vi "S8300E_SATA_HDD_Model_WIH.vi"() -> ()   [LabVIEW 2011]
panel:
  out "PRELOG2":string
  out "PRELOG1":string
  out "SATA_HDD_NUM":string
  out "CMDList":cluster{string, string, string}[](array[cluster])
  out "log msg":string
  out "VISA resource name out":refnum<visa-resource-name>
  out "BEGIN TIME":u32
  out "進行狀況":string
  # "2015-6-1"
  # "S8300E SATA  HDD Model Test(接UART COM9)"
  # "Error Code:SATA-HDD"
  # "Please insert the correct HDD Drive for Shipment\n請插入正確的出貨硬碟 (Model numer 需正確輸入於特定文檔)"
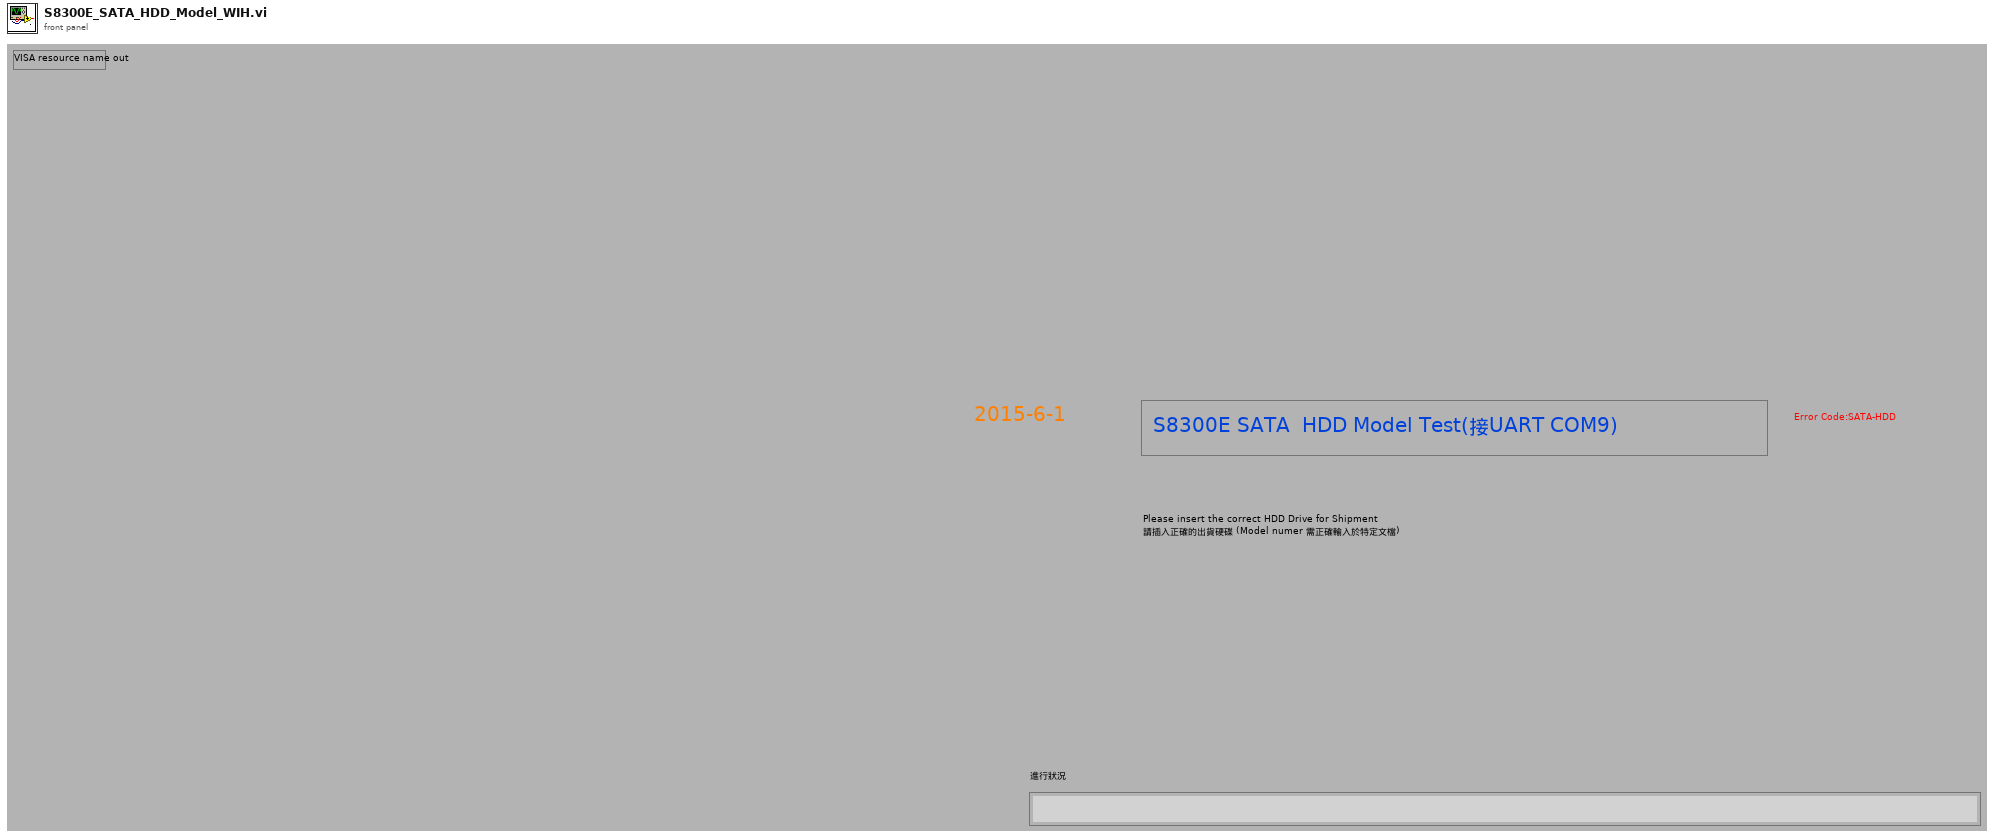
[diagram p1: front panel]
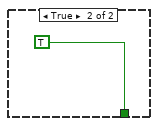
[diagram p7: hidden frame]
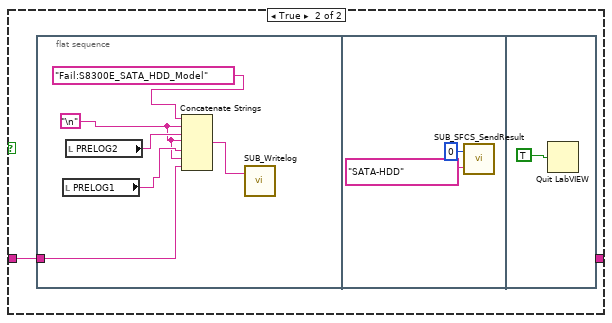
[diagram p8: hidden frame]
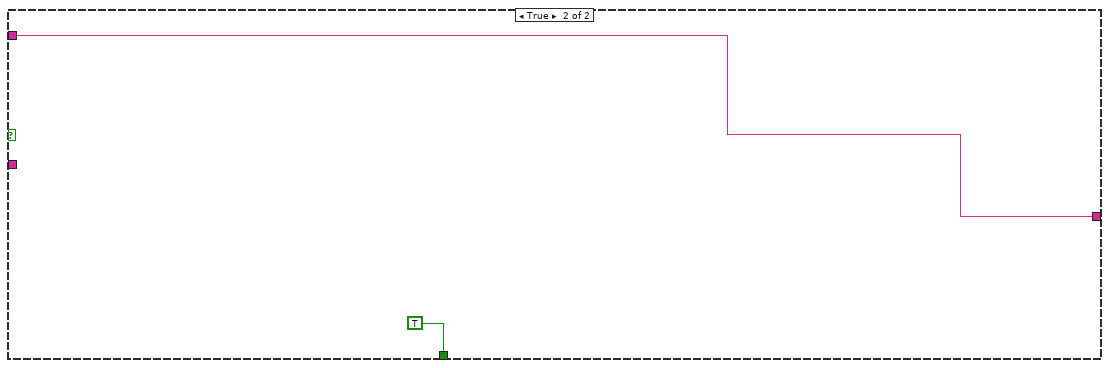
[diagram p9: hidden frame]
diagram:
  n1 = flat-sequence {
    frame #0 {
      n2 = Tick Count (ms)() -> (millisecond timer value=→"BEGIN TIME":u32)
    }
    frame #1 {
      n3 = property on="進行狀況" class="Str"("Blinking"=TRUE) -> ()  [unwired: 2 in, 2 out]
      "進行狀況" <- "進入測試準備中...." ("進行狀況")
    }
    frame #2 {
      n4 = call "SUB_SearchFile_inFolder.vi"("Search Filename in Folder"="S8300E_sfcs_misc.txt") -> ("File Existing True/Flase"=w4:bool)  [unwired: 1 in]
      n5 = case shown="False" w4 {
        frame False {
          n6 = flat-sequence {
            frame #0 {
              n7 = call "Display Message to User"() -> ()  [unwired: 10 in, 2 out]
            }
            frame #1 {
              n8 = call "SUB_Writelog.vi"("Pass/Fail"="Fail:S8300E_SATA_HDD_Model") -> ()  [unwired: 2 in]
            }
            frame #2 {
              n9 = Quit LabVIEW(quit? (T)=TRUE) -> ()
            }
          }
        }
        frame True {
        }
      }
    }
    frame #3 {
      n10 = call "SUB_Read_specifFile.vi"("name or relative path"="S8300E_sfcs_misc.txt" ("Search Filename in Folder")) -> ("text"=w11:string)  [unwired: 1 in, 1 out]
      n11 = call "SUB_FindSpecificString.vi"("Find this String"="UUT_SATA_HDD_MODEL=", "String data"=w11) -> ("before \"; \" string"=→"SATA_HDD_NUM":string, "Found"=w9:bool)  [unwired: 2 in]
      n12 = case shown="False" w9 {
        frame False {
          n13 = flat-sequence {
            frame #0 {
              n14 = call "Display Message to User2"() -> ()  [unwired: 10 in, 2 out]
            }
            frame #1 {
              n15 = call "SUB_Writelog.vi"("Pass/Fail"="Fail:S8300E_SATA_HDD_Model") -> ()  [unwired: 2 in]
            }
            frame #2 {
              n16 = Quit LabVIEW(quit? (T)=TRUE) -> ()
            }
          }
        }
        frame True {
        }
      }
    }
    frame #4 {
      n17 = local read "SATA_HDD_NUM"() -> (w16:string)
      n18 = Concatenate Strings("PASSED=", w16) -> (w15:string)
      n19 = Concatenate Strings("./sata.sh -m 1", "\r") -> (w21:string)
      n20 = Bundle(w21, w15, "Checking SATA  HDD Mdel Number") -> (w19:cluster{string, string, string})  [unwired: 1 in]
      n21 = Build Array(w19) -> (→"CMDList":cluster{string, string, string}[])
    }
    frame #5 {
      n22 = call "SUB_COM1_CLOSE.vi"("VISA resource name"=refnum<visa-resource-name> "COM9") -> ()  [unwired: 3 in]
    }
    frame #6 {
      n23 = case shown="True" TRUE {
        frame False {
        }
        frame True {
          n24 = call "SUB_COM9_INIT.vi"("baud rate"=u32 115200) -> ("VISA resource name out"=w29:refnum<visa-resource-name>)  [unwired: 1 in, 1 out]
          "VISA resource name out" <- w29
          n25 = call "SUB_COM1Wrt.vi"("VISA resource name"=w29, "write buffer"="\r") -> ("duplicate VISA resource name"=w26:refnum<visa-resource-name>)  [unwired: 1 in, 1 out]
          n26 = call "SUB_ContinueCom1Read.vi"("Numeric"=1200, "duplicate VISA resource name 2"=w26) -> ()  [unwired: 1 in, 3 out]
        }
      }
    }
    frame #7 {
      n27 = case shown="True" TRUE {
        frame False {
        }
        frame True {
          n28 = while {
            stop <- w41 stop-if-true
            n29 = local read "VISA resource name out"() -> (w32:refnum<visa-resource-name>)
            n30 = call "SUB_ContinueCom1Read.vi"("Numeric"=1200, "duplicate VISA resource name 2"=w32) -> ("duplicate VISA resource name"=w33:refnum<visa-resource-name>)  [unwired: 1 in, 2 out]
            n31 = call "SUB_COM1Wrt.vi"("VISA resource name"=w33, "write buffer"="\r") -> ("duplicate VISA resource name"=w40:refnum<visa-resource-name>)  [unwired: 1 in, 1 out]
            n32 = Tick Count (ms)() -> (millisecond timer value=w39:u32)
            n33 = call "SUB_READ_COM1_FindString_timeout.vi"("Find this String"="s8300e_func_test#", "Timeout Seccond"=3.0, "Begin time"=w39, "duplicate VISA resource name 2"=w40) -> ("Output String"=w35:string, "Found String"=w36:bool)  [unwired: 1 in, 1 out]
            n34 = case shown="False" w36 {
              tunnel: [w47 TRUE] -> w41
              tunnel: w35 -> [w44 _]
              frame False {
                w46 = "UART無正確反應!需有S8300E字串" ("Status")
                n35 = call "SUB_YESNO.vi"("Debug View"=w44, "Status"=w46) -> ("yes/no"=w50:enum32{"No Selection", "Yes", "No", "None"})  [unwired: 1 in]
                n36 = Concatenate Strings(w46, "\n", w44) -> (w43:string)
                n37 = Equal?(x=w50, y=enum32{"No Selection", "Yes", "No", "None"}."No") -> (x = y?=w48:bool)
                n38 = case shown="True" w48 {
                  tunnel: [_ w52] -> w47
                  tunnel: w43 -> [_ w51]
                  frame False {
                  }
                  frame True {
                    n39 = flat-sequence {
                      tunnel: w51 -> [w54]
                      tunnel: [w59] -> w52
                      frame #0 {
                        n40 = Concatenate Strings("Fail:S8300E_SATA_HDD_Model" ("Pass/Fail"), "\n", w54) -> (w53:string)
                        n41 = call "SUB_Writelog.vi"("Pass/Fail"=w53) -> ()  [unwired: 2 in]
                      }
                      frame #1 {
                        n42 = call "SUB_SFCS_SendResult.vi"("ErrorCode"="UART", "PASS_Fail (1/0)"=i8 0) -> ()  [unwired: 1 out]
                      }
                      frame #2 {
                        w59 = TRUE ("quit? (T)")
                        n43 = Quit LabVIEW(quit? (T)=w59) -> ()
                      }
                    }
                  }
                }
              }
              frame True {
              }
            }
          }
        }
      }
    }
    frame #8 {
      n44 = local write "log msg"("") -> ()
    }
    frame #9 {
      n45 = local read "CMDList"() -> (w62:cluster{string, string, string}[])
      n46 = Array Size(array=w62) -> (size(s)=w65:i32)
      n47 = for {
        N: w65 -> [_]
        shift-right: [w67] -> w63
        shift-left: "" -> [w66]
        i -> [w70]
        n48 = while {
          tunnel: w70 -> [w90]
          shift-right: [w80] -> w68
          shift-left: "" -> [w79]
          stop <- w85 stop-if-true
          n49 = local read "VISA resource name out"() -> (w72:refnum<visa-resource-name>)
          n50 = local read "CMDList"() -> (w83:cluster{string, string, string}[])
          n51 = Index Array(array=w83, index=w90) -> (element=w84:cluster{string, string, string})
          n52 = call "SUB_ContinueCom1Read.vi"("Numeric"=1200, "duplicate VISA resource name 2"=w72) -> ("duplicate VISA resource name"=w71:refnum<visa-resource-name>)  [unwired: 1 in, 2 out]
          n53 = Unbundle(w84) -> (w78:string, w81:string, w82:string)
          n54 = call "SUB_COM1Wrt.vi"("VISA resource name"=w71, "write buffer"=w78) -> ("duplicate VISA resource name"=w89:refnum<visa-resource-name>)  [unwired: 1 in, 1 out]
          n55 = Tick Count (ms)() -> (millisecond timer value=w88:u32)
          n56 = call "SUB_READ_COM1_FindString_timeout.vi"("Find this String"=w81, "Timeout Seccond"=3.0, "Begin time"=w88, "duplicate VISA resource name 2"=w89) -> ("Output String"=w76:string, "Found String"=w86:bool)  [unwired: 1 in, 1 out]
          n57 = local write "進行狀況"(w82) -> ()
          n58 = Concatenate Strings(w78, "\n", w76) -> (w75:string)
          n59 = case shown="False" w86 {
            tunnel: [_ TRUE] -> w85
            tunnel: w76 -> [w99 _]
            tunnel: w75 -> [w93 w111]
            tunnel: [w91 w111] -> w74
            frame False {
              w95 = "SATA測試失敗 or 型號不符合!有插入正確出貨SATA DRIVE" ("string")
              n60 = Concatenate Strings(w95, "\n", w93) -> (w92:string)
              n61 = call "SUB_YESNO.vi"("Debug View"=w99, "Status"=w95) -> ("yes/no"=w98:enum32{"No Selection", "Yes", "No", "None"})  [unwired: 1 in]
              n62 = Equal?(x=w98, y=enum32{"No Selection", "Yes", "No", "None"}."No") -> (x = y?=w96:bool)
              n63 = case shown="False" w96 {
                tunnel: w92 -> [w100 w101]
                tunnel: [w100 _] -> w91
                frame False {
                }
                frame True {
                  n64 = flat-sequence {
                    tunnel: w101 -> [w103]
                    frame #0 {
                      w104 = "\n"
                      n65 = local read "PRELOG1"() -> (w105:string)
                      n66 = local read "PRELOG2"() -> (w106:string)
                      n67 = Concatenate Strings("Fail:S8300E_SATA_HDD_Model" ("Pass/Fail"), w104, w106, w104, w105, w104, w103) -> (w102:string)
                      n68 = call "SUB_Writelog.vi"("Pass/Fail"=w102) -> ()  [unwired: 2 in]
                    }
                    frame #1 {
                      n69 = call "SUB_SFCS_SendResult.vi"("ErrorCode"="SATA-HDD", "PASS_Fail (1/0)"=i8 0) -> ()  [unwired: 1 out]
                    }
                    frame #2 {
                      n70 = Quit LabVIEW(quit? (T)=TRUE) -> ()
                    }
                  }
                }
              }
            }
            frame True {
            }
          }
          n71 = Concatenate Strings(w79, w74) -> (w80:string)
          "PRELOG1" <- w80
        }
        n72 = Concatenate Strings(w66, w68) -> (w67:string)
        "PRELOG2" <- w67
      }
      "log msg" <- w63
    }
    frame #10 {
      n73 = call "SUB_COM1_CLOSE.vi"("VISA resource name"=refnum<visa-resource-name> "COM9") -> ()  [unwired: 3 in]
    }
    frame #11 {
      w116 = "***Not Good ***" ("replace string (\"\")")
      n74 = local read "log msg"() -> (w120:string)
      n75 = local read "BEGIN TIME"() -> (w125:u32)
      n76 = Tick Count (ms)() -> (millisecond timer value=w124:u32)
      n77 = call "SUB_CAL_TESTTIME.vi"("Test Item name"="S8300E_SATA_HDD_Model", "Stop tick time"=w124, "Start tick time"=w125) -> ("Test Time output"=w122:string)  [unwired: 2 in]
      n78 = Concatenate Strings("Pass:S8300E_SATA_HDD_Model", "\n", w120, w122) -> (w115:string)
      n79 = call "SUB_SEARCH_REPLACE_STR.vi"("replace string (\"\")"=w116, "search string"="FAILED", "input string"=w115) -> ("result string"=w118:string)  [unwired: 2 in]
      n80 = call "SUB_SEARCH_REPLACE_STR.vi"("replace string (\"\")"=w116, "search string"="FAIL", "input string"=w118) -> ("result string"=w114:string)  [unwired: 2 in]
      n81 = call "SUB_Writelog.vi"("Pass/Fail"=w114) -> ()  [unwired: 2 in]
    }
    frame #12 {
      n82 = Request Deallocation(TRUE ("flag")) -> ()
    }
    frame #13 {
      n83 = Quit LabVIEW(quit? (T)=TRUE ("stop? (T)")) -> ()
    }
  }
